vi "Untitled 1.vi"(8 "error in (no error)":errorcluster, 11 "DAQOrcaFlash in":refnum<class "DAQOrcaFlash.lvclass">) -> (0 "error out":errorcluster, 3 "DAQOrcaFlash out":refnum<class "DAQOrcaFlash.lvclass">)   [LabVIEW 2012, in "DAQOrcaFlash.lvclass"]
uses:
  DAQOrcaFlash.lvclass
  dependencies/LabTIFF/LabTIFF/Opening Purpose.ctl
  <vilib>/vision/NI_Vision_Development_Module.lvlib
panel:
  out "ms to calculate trace":u32
  out "ms for frame loop before display":u32
  out "ms for one frame loop":u32
  out "ms to read frame into imaq":u32
  out "ms to calculate running av":u32
  out "after downsampling":dbl
  out "baseline number":i32
  out "min trace":sgl
  out "max tace":sgl
  out "max baseline":sgl
  out "min baseline":sgl
  out "min frame":sgl
  out "max frame":sgl
  out "max running sum":sgl
  out "min running sum":sgl
  out "min div":sgl
  out "max div":sgl
  out "Total Frames":i32
  out "baseline counter":i32
  out "downsampling counter":i32
  out "part of baseline":bool
  out "calculate average":bool
  in  "cxd folder Path":path
  # "of"
  # "of"
  # "cxd temporally downsampled"
  # "baseline"
  # "trace"
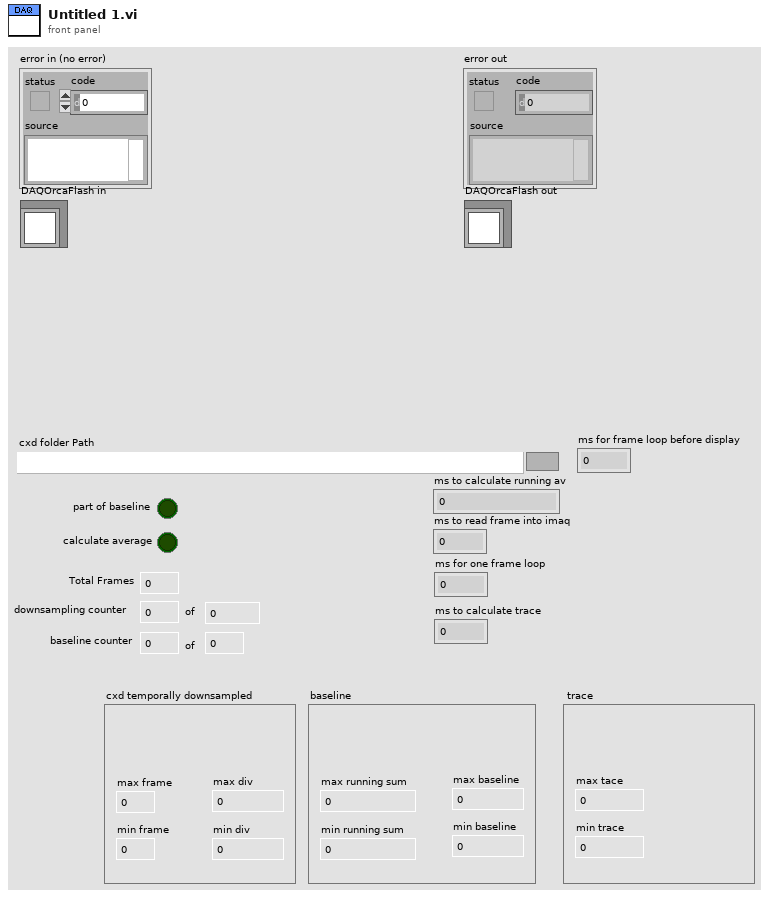
[diagram p1: front panel]
types:
  T1 = typedef "Opening Purpose.ctl" = enum16{"Read", "Write"}
  T2 = typedef "Image Type" = u32
  T3 = typedef "IMAQ Image.ctl" = refnum<image>
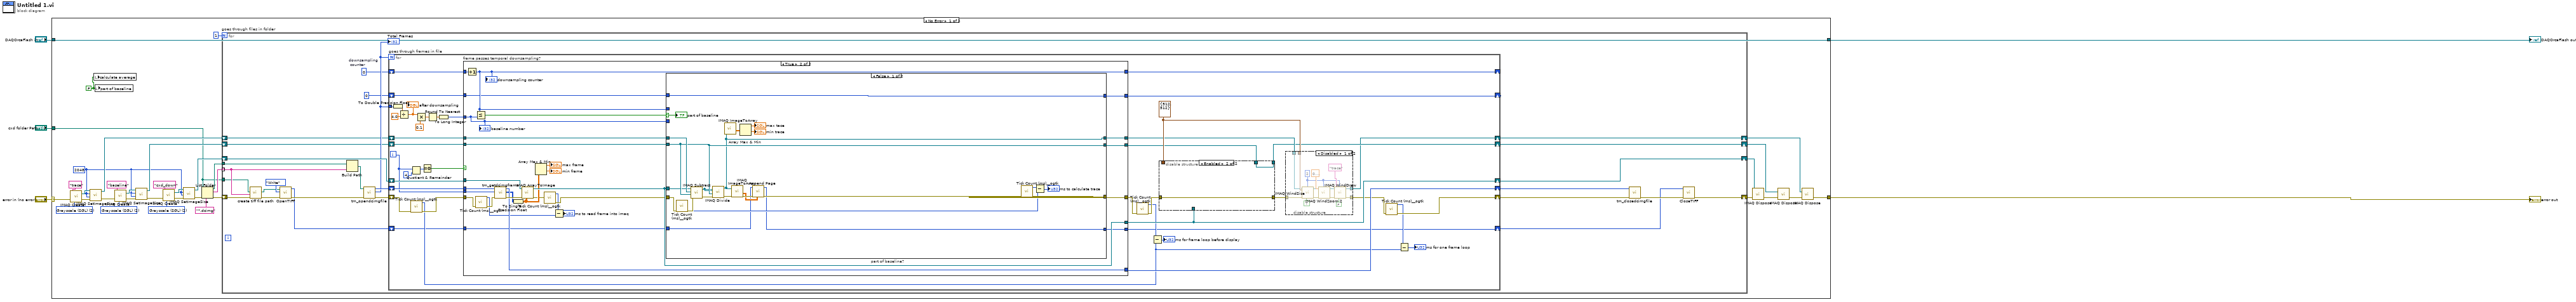
[diagram p0: block diagram]
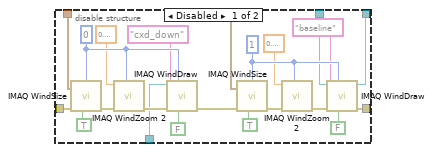
[diagram p3: hidden frame]
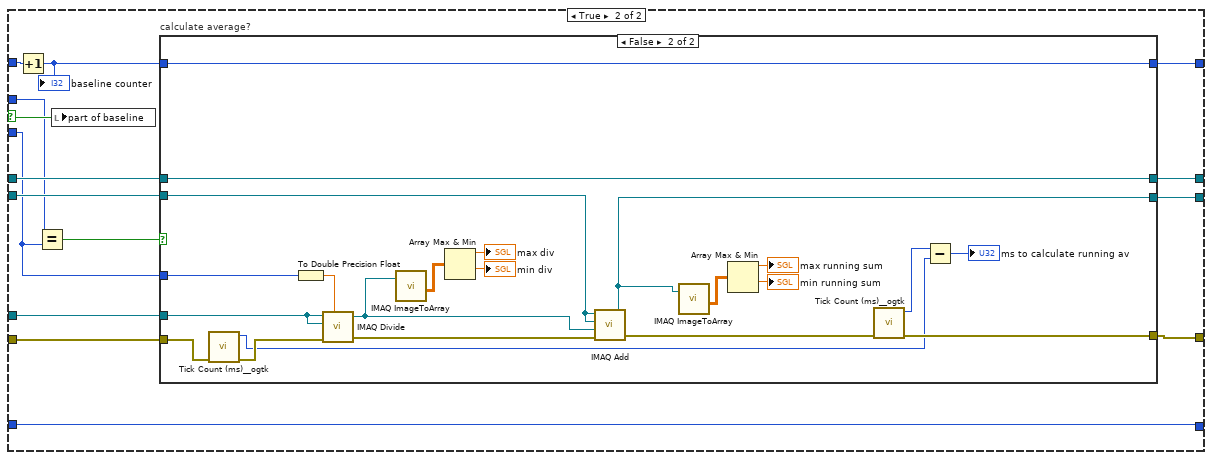
[diagram p5: hidden frame]
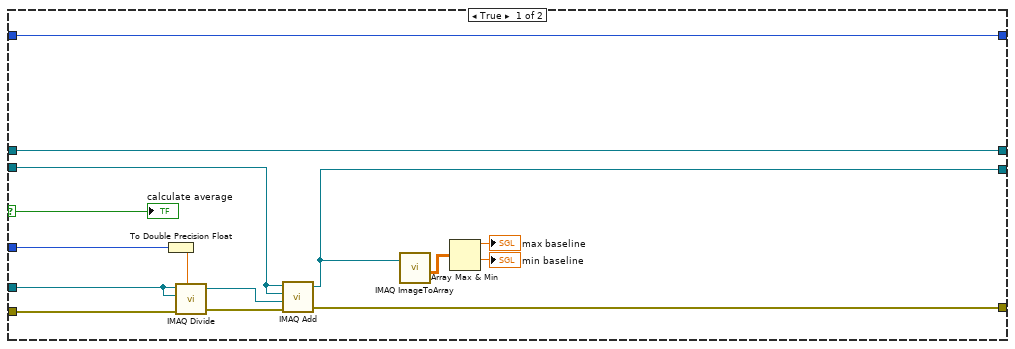
[diagram p6: hidden frame]
diagram:
  n1 = case shown="No Error" "error in (no error)" {
    selector: "error in (no error)" -> [w22 w259]
    tunnel: [w26 w259] -> w4
    tunnel: [w40 w258] -> w2
    tunnel: "DAQOrcaFlash in" -> [w40 w258]
    tunnel: "cxd folder Path" -> [w6 _]
    frame No Error {
      w7 = FALSE ("part of baseline")
      w8 = 2048 ("X Resolution")
      w24 = T2 2 items=["Grayscale (U8)", "Grayscale (I16)", "Grayscale (SGL)", "Complex (CSG)", "RGB (U32)", "HSL (U32)", "RGB (U64)", "Grayscale (U16)"] ("Image Type")
      w29 = T2 2 items=["Grayscale (U8)", "Grayscale (I16)", "Grayscale (SGL)", "Complex (CSG)", "RGB (U32)", "HSL (U32)", "RGB (U64)", "Grayscale (U16)"] ("Image Type")
      w34 = T2 2 items=["Grayscale (U8)", "Grayscale (I16)", "Grayscale (SGL)", "Complex (CSG)", "RGB (U32)", "HSL (U32)", "RGB (U64)", "Grayscale (U16)"] ("Image Type")
      n2 = call "IMAQ Create"("Image Name"="trace", "Image Type"=w24, "error in (no error)"=w22) -> ("New Image"=w14:T3, "error out"=w20:errorcluster)  [unwired: 2 in]
      n3 = call "IMAQ SetImageSize"("error in (no error)"=w20, "Y Resolution"=w8, "X Resolution"=w8, "Image"=w14) -> ("error out"=w19:errorcluster, "Image Out"=w13:T3)  [unwired: 1 in]
      n4 = local write "calculate average"(w7) -> ()
      n5 = local write "part of baseline"(w7) -> ()
      n6 = call "IMAQ Create"("Image Name"="baseline", "Image Type"=w29, "error in (no error)"=w19) -> ("New Image"=w12:T3, "error out"=w18:errorcluster)  [unwired: 2 in]
      n7 = call "IMAQ SetImageSize"("error in (no error)"=w18, "Y Resolution"=w8, "X Resolution"=w8, "Image"=w12) -> ("error out"=w17:errorcluster, "Image Out"=w11:T3)  [unwired: 1 in]
      n8 = call "IMAQ Create"("Image Name"="cxd_down", "Image Type"=w34, "error in (no error)"=w17) -> ("New Image"=w10:T3, "error out"=w16:errorcluster)  [unwired: 2 in]
      n9 = call "IMAQ SetImageSize"("error in (no error)"=w16, "Y Resolution"=w8, "X Resolution"=w8, "Image"=w10) -> ("error out"=w15:errorcluster, "Image Out"=w9:T3)  [unwired: 1 in]
      n10 = List Folder(path=w6, pattern="*.dcimg", error in=w15) -> (path out=w35:path, filenames=w36:string[], error out=w37:errorcluster)  [unwired: 1 in, 1 out]
      n11 = for "goes through files in folder" {
        N: 1 -> [_]
        tunnel: w36 -> [w48] mode=indexing
        tunnel: w35 -> [w47]
        shift-right: [w43] -> w32
        shift-left: w37 -> [w50]
        shift-right: [w62] -> w31
        shift-left: w9 -> [w63]
        shift-right: [w56] -> w25
        shift-left: w11 -> [w57]
        shift-right: [w53] -> w21
        shift-left: w13 -> [w54]
        tunnel: w6 -> [w41]
        w58 = 0  # downsampling  counter
        n12 = call "create tiff file path.vi"("error in (no error)"=w50, "dcimg name"=w48, "cxd folder Path"=w41) -> ("error IO"=w49:errorcluster, "tiff file path"=w46:path)  [unwired: 6 in, 1 out]
        n13 = call "OpenTIFF.vi"("error in (no error)"=w49, "Opening Purpose"=Opening_Purpose."Write", "File Path"=w46) -> ("error out"=w51:errorcluster, "TIFF File Ref"=w45:i32)  [unwired: 7 in]
        n14 = Build Path(base path=w47, name or relative path=w48) -> (appended path=w66:path)
        n15 = call <userlib>:"tm_opendcimgfile.vi"("error in (no error)"=w51, "Path"=w66) -> ("error out"=w65:errorcluster, "Total Frames"=w59:i32, "File Handle"=w64:u32)  [unwired: 7 in]
        "Total Frames" <- w59
        n16 = for "goes through frames in file" {
          N: w59 -> [_]
          shift-right: [w76] -> w60
          shift-left: w65 -> [w79]
          shift-right: [w83] -> w62
          shift-left: w63 -> [w103]
          shift-right: [w101] -> w61
          shift-left: w64 -> [w107]
          tunnel: w59 -> [w98]
          shift-right: [w94] -> _
          shift-left: w58 -> [w92]
          shift-right: [w82] -> w56
          shift-left: w57 -> [w90]
          shift-right: [w88] -> _
          shift-left: 0 -> [w89]
          shift-right: [w81] -> w53
          shift-left: w54 -> [w87]
          shift-right: [w67] -> w42
          shift-left: w45 -> [w68]
          i -> [w102]
          w86 = cluster{"Width":i32, "Height":i32} {"Width"=512, "Height"=512} ("Width & Height")
          n17 = To Double Precision Float(number=w98) -> (double precision float=w100:dbl)
          n18 = Divide(x=w100, y=4.0) -> (x/y=w95:dbl)
          "after downsampling" <- w95
          n19 = Quotient & Remainder(x=w102, y=4) -> (x-y*floor(x/y)=w105:i32)  [unwired: 1 out]
          n20 = call <userlib>:"Tick Count (ms)__ogtk.vi"("error in (no error)"=w79) -> ("error out"=w78:errorcluster, "millisecond timer value"=w71:u32)  [unwired: 9 in]
          n21 = Multiply(x=w95, y=0.1) -> (x*y=w97:dbl)
          n22 = Equal To 0?(x=w105) -> (x = 0?=w104:bool)
          n23 = Round To Nearest(number=w97) -> (nearest integer value=w93:dbl)
          n24 = To Long Integer(number=w93) -> (32bit integer=w91:i32)
          n25 = case "frame passes temporal downsampling?" shown="True" w104 {
            tunnel: w78 -> [w152 w161]
            tunnel: w107 -> [w151 w182]
            tunnel: w103 -> [w146 w180]
            tunnel: [w152 w175] -> w72
            tunnel: [w151 w179] -> w101
            tunnel: w102 -> [_ w178]
            tunnel: w92 -> [w150 w177]
            tunnel: [w150 w171] -> w94
            tunnel: w91 -> [_ w172]
            tunnel: w90 -> [w148 w174]
            tunnel: [w148 w173] -> w84
            tunnel: w89 -> [w149 w170]
            tunnel: [w149 w169] -> w88
            tunnel: w87 -> [w147 w168]
            tunnel: [w147 w167] -> w85
            tunnel: [w146 w165] -> w83
            tunnel: w68 -> [w145 w154]
            tunnel: [w145 w153] -> w67
            frame False {
            }
            frame True {
              n26 = Increment(x=w177) -> (x+1=w171:i32)
              "downsampling counter" <- w171
              n27 = Less Or Equal?(x=w171, y=w172) -> (x <= y?=w176:bool)
              n28 = call <userlib>:"Tick Count (ms)__ogtk.vi"("error in (no error)"=w161) -> ("error out"=w160:errorcluster, "millisecond timer value"=w156:u32)  [unwired: 9 in]
              n29 = call <userlib>:"tm_getdcimgframe.vi"("error in (no error)"=w160, "Frame Index"=w178, "File Handle in"=w182) -> ("error out"=w181:errorcluster, "Data"=w166:u16[][], "File Handle out"=w179:u32)  [unwired: 5 in, 1 out]
              n30 = To Single Precision Float(number=w166) -> (single precision float=w164:sgl[][])
              n31 = call "IMAQ ArrayToImage"("Image Pixels (Float)"=w164, "error in (no error)"=w181, "Image"=w180) -> ("error out"=w159:errorcluster, "Image Out"=w165:T3)  [unwired: 7 in]
              n32 = Array Max & Min(array=w164) -> (max value=→"max frame":sgl, min value=→"min frame":sgl)  [unwired: 2 out]
              n33 = call <userlib>:"Tick Count (ms)__ogtk.vi"("error in (no error)"=w159) -> ("error out"=w158:errorcluster, "millisecond timer value"=w157:u32)  [unwired: 9 in]
              n34 = Subtract(x=w157, y=w156) -> (x-y=→"ms to read frame into imaq":u32)
              n35 = case "part of baseline?" shown="False" w176 {
                selector: w176 -> [w200 w209]
                tunnel: w158 -> [w194 w220]
                tunnel: w165 -> [w201 w216]
                tunnel: [w195 w219] -> w175
                tunnel: w174 -> [w202 w218]
                tunnel: [w202 w217] -> w173
                tunnel: w172 -> [_ w208]
                tunnel: w171 -> [_ w207]
                tunnel: w170 -> [w205 w214]
                tunnel: [w205 w212] -> w169
                tunnel: w168 -> [w204 w211]
                tunnel: [w188 w210] -> w167
                tunnel: w154 -> [w184 w206]
                tunnel: [w183 w206] -> w153
                frame False {
                  n36 = call <userlib>:"Tick Count (ms)__ogtk.vi"("error in (no error)"=w194) -> ("error out"=w193:errorcluster, "millisecond timer value"=w191:u32)  [unwired: 9 in]
                  n37 = call "IMAQ Subtract"("Image Src A"=w201, "Image Dst"=w204, "Image Src B"=w202, "error in (no error)"=w193) -> ("Image Dst Out"=w199:T3, "error out"=w203:errorcluster)  [unwired: 3 in]
                  n38 = call "IMAQ Divide"("Image Src A"=w199, "Image Dst"=w199, "Image Src B"=w202, "error in (no error)"=w203) -> ("Image Dst Out"=w188:T3, "error out"=w189:errorcluster)  [unwired: 3 in]
                  n39 = call "IMAQ ImageToArray"("Image"=w188) -> ("Image Pixels (Float)"=w198:sgl[][])  [unwired: 3 in, 4 out]
                  n40 = call "IMAQ ImageToArray"("error in (no error)"=w189, "Image"=w188) -> ("Image Pixels (Float)"=w185:sgl[][], "error out"=w187:errorcluster)  [unwired: 2 in, 3 out]
                  n41 = Array Max & Min(array=w198) -> (max value=→"max tace":sgl, min value=→"min trace":sgl)  [unwired: 2 out]
                  n42 = call "Append Page.vi"("Float32 Image"=w185, "error in (no error)"=w187, "TIFF File Ref"=w184) -> ("error out"=w186:errorcluster, "TIFF File Ref out"=w183:i32)  [unwired: 7 in]
                  n43 = call <userlib>:"Tick Count (ms)__ogtk.vi"("error in (no error)"=w186) -> ("error out"=w195:errorcluster, "millisecond timer value"=w192:u32)  [unwired: 9 in]
                  n44 = Subtract(x=w192, y=w191) -> (x-y=→"ms to calculate trace":u32)
                  "part of baseline" <- w200
                }
                frame True {
                  n45 = Increment(x=w214) -> (x+1=w213:i32)
                  "baseline counter" <- w213
                  n46 = Equal?(x=w207, y=w208) -> (x = y?=w215:bool)
                  n47 = local write "part of baseline"(w209) -> ()
                  n48 = case "calculate average?" shown="False" w215 {
                    selector: w215 -> [w231 _]
                    tunnel: w220 -> [w230 w248]
                    tunnel: [w225 w245] -> w219
                    tunnel: w218 -> [w234 w255]
                    tunnel: [w221 w249] -> w217
                    tunnel: w216 -> [w229 w251]
                    tunnel: w213 -> [w233 w257]
                    tunnel: [w233 w257] -> w212
                    tunnel: w211 -> [w235 w256]
                    tunnel: [w235 w256] -> w210
                    tunnel: w208 -> [w228 w252]
                    frame True {
                      n49 = To Double Precision Float(number=w228) -> (double precision float=w232:dbl)
                      n50 = call "IMAQ Divide"("Image Src A"=w229, "Constant"=w232, "Image Dst"=w229, "error in (no error)"=w230) -> ("Image Dst Out"=w226:T3, "error out"=w227:errorcluster)  [unwired: 3 in]
                      n51 = call "IMAQ Add"("Image Src A"=w234, "Image Dst"=w234, "Image Src B"=w226, "error in (no error)"=w227) -> ("Image Dst Out"=w221:T3, "error out"=w225:errorcluster)  [unwired: 3 in]
                      n52 = call "IMAQ ImageToArray"("Image"=w221) -> ("Image Pixels (Float)"=w222:sgl[][])  [unwired: 3 in, 4 out]
                      n53 = Array Max & Min(array=w222) -> (max value=→"max baseline":sgl, min value=→"min baseline":sgl)  [unwired: 2 out]
                      "calculate average" <- w231
                    }
                    frame False {
                      n54 = call <userlib>:"Tick Count (ms)__ogtk.vi"("error in (no error)"=w248) -> ("error out"=w247:errorcluster, "millisecond timer value"=w236:u32)  [unwired: 9 in]
                      n55 = To Double Precision Float(number=w252) -> (double precision float=w253:dbl)
                      n56 = call "IMAQ Divide"("Image Src A"=w251, "Constant"=w253, "Image Dst"=w251, "error in (no error)"=w247) -> ("Image Dst Out"=w250:T3, "error out"=w254:errorcluster)  [unwired: 3 in]
                      n57 = call "IMAQ ImageToArray"("Image"=w250) -> ("Image Pixels (Float)"=w241:sgl[][])  [unwired: 3 in, 4 out]
                      n58 = Array Max & Min(array=w241) -> (max value=→"max div":sgl, min value=→"min div":sgl)  [unwired: 2 out]
                      n59 = call "IMAQ Add"("Image Src A"=w255, "Image Dst"=w255, "Image Src B"=w250, "error in (no error)"=w254) -> ("Image Dst Out"=w249:T3, "error out"=w246:errorcluster)  [unwired: 3 in]
                      n60 = call "IMAQ ImageToArray"("Image"=w249) -> ("Image Pixels (Float)"=w240:sgl[][])  [unwired: 3 in, 4 out]
                      n61 = Array Max & Min(array=w240) -> (max value=→"max running sum":sgl, min value=→"min running sum":sgl)  [unwired: 2 out]
                      n62 = call <userlib>:"Tick Count (ms)__ogtk.vi"("error in (no error)"=w246) -> ("error out"=w245:errorcluster, "millisecond timer value"=w237:u32)  [unwired: 9 in]
                      n63 = Subtract(x=w237, y=w236) -> (x-y=→"ms to calculate running av":u32)
                    }
                  }
                }
              }
              "baseline number" <- w172
            }
          }
          n64 = call <userlib>:"Tick Count (ms)__ogtk.vi"("error in (no error)"=w72) -> ("error out"=w73:errorcluster, "millisecond timer value"=w70:u32)  [unwired: 9 in]
          n65 = Subtract(x=w70, y=w71) -> (x-y=→"ms for frame loop before display":u32)
          n66 = disable-structure shown="Enabled" {
            disable-tunnel: w86 -> [w128 _]
            disable-tunnel: w84 -> [w127 w143]
            disable-tunnel: w83 -> [w126 _]
            disable-tunnel: [w125 w143] -> w82
            disable-tunnel: [w123 w144] -> w80
            disable-tunnel: w73 -> [w122 w144]
            frame Disabled {
              w133 = 1 ("Window Number")
              w139 = 0 ("Window Number")
              n67 = call "IMAQ WindSize"("error in (no error)"=w122, "Get/Set Status? (Set)"=TRUE, "Width & Height"=w128, "Window Number"=w139) -> ("error out"=w141:errorcluster)  [unwired: 2 in, 2 out]
              n68 = call "IMAQ WindZoom 2"("Window Number (0...15)"=w139, "error in (no error)"=w141, "Zoom Factor"=sgl 0.2) -> ("error out"=w140:errorcluster)  [unwired: 5 in, 3 out]
              n69 = call "IMAQ WindDraw"("Resize to Image Size? (Y)"=FALSE, "Window Number (0...15)"=w139, "error in (no error)"=w140, "Title"="cxd_down", "Image"=w126) -> ("error out"=w124:errorcluster)  [unwired: 5 in, 1 out]
              n70 = call "IMAQ WindSize"("error in (no error)"=w124, "Get/Set Status? (Set)"=TRUE, "Width & Height"=w128, "Window Number"=w133) -> ("error out"=w135:errorcluster)  [unwired: 2 in, 2 out]
              n71 = call "IMAQ WindZoom 2"("Window Number (0...15)"=w133, "error in (no error)"=w135, "Zoom Factor"=sgl 0.2) -> ("error out"=w134:errorcluster)  [unwired: 5 in, 3 out]
              n72 = call "IMAQ WindDraw"("Resize to Image Size? (Y)"=FALSE, "Window Number (0...15)"=w133, "error in (no error)"=w134, "Title"="baseline", "Image"=w127) -> ("error out"=w123:errorcluster, "Image Out (duplicate)"=w125:T3)  [unwired: 5 in]
            }
            frame Enabled {
            }
          }
          n73 = disable-structure shown="Disabled" {
            disable-tunnel: w86 -> [w112 _]
            disable-tunnel: w85 -> [w111 w120]
            disable-tunnel: [w110 w120] -> w81
            disable-tunnel: w80 -> [w109 w121]
            disable-tunnel: [w108 w121] -> w77
            frame Disabled {
              w116 = 2 ("Window Number")
              n74 = call "IMAQ WindSize"("error in (no error)"=w109, "Get/Set Status? (Set)"=TRUE, "Width & Height"=w112, "Window Number"=w116) -> ("error out"=w114:errorcluster)  [unwired: 2 in, 2 out]
              n75 = call "IMAQ WindZoom 2"("Window Number (0...15)"=w116, "error in (no error)"=w114, "Zoom Factor"=sgl 0.2) -> ("error out"=w115:errorcluster)  [unwired: 5 in, 3 out]
              n76 = call "IMAQ WindDraw"("Resize to Image Size? (Y)"=FALSE, "Window Number (0...15)"=w116, "error in (no error)"=w115, "Title"="trace", "Image"=w111) -> ("error out"=w108:errorcluster, "Image Out (duplicate)"=w110:T3)  [unwired: 5 in]
            }
            frame Enabled {
            }
          }
          n77 = call <userlib>:"Tick Count (ms)__ogtk.vi"("error in (no error)"=w77) -> ("error out"=w76:errorcluster, "millisecond timer value"=w75:u32)  [unwired: 9 in]
          n78 = Subtract(x=w75, y=w71) -> (x-y=→"ms for one frame loop":u32)
        }
        n79 = call <userlib>:"tm_closedcimgfile.vi"("error in (no error)"=w60, "File Handle"=w61) -> ("error out"=w44:errorcluster)  [unwired: 9 in]
        n80 = call "CloseTIFF.vi"("error in (no error)"=w44, "TIFF File Ref"=w42) -> ("error out"=w43:errorcluster)  [unwired: 9 in]
      }
      n81 = call "IMAQ Dispose"("Image"=w31, "error in (no error)"=w32) -> ("error out"=w27:errorcluster)  [unwired: 4 in]
      n82 = call "IMAQ Dispose"("Image"=w25, "error in (no error)"=w27) -> ("error out"=w28:errorcluster)  [unwired: 4 in]
      n83 = call "IMAQ Dispose"("Image"=w21, "error in (no error)"=w28) -> ("error out"=w26:errorcluster)  [unwired: 4 in]
    }
    frame Error {
    }
  }
  "error out" <- w4
  "DAQOrcaFlash out" <- w2
